vi "thermometer_prac2.vi"() -> ()   [LabVIEW 2020]
panel:
  in  "Skala temperatury":bool
  out "Temperatura [F]":dbl(slide) scale=0.0..100.0
  out "Temperatura [C]":dbl(slide) scale=0.0..100.0
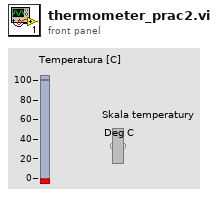
[diagram p1: front panel]
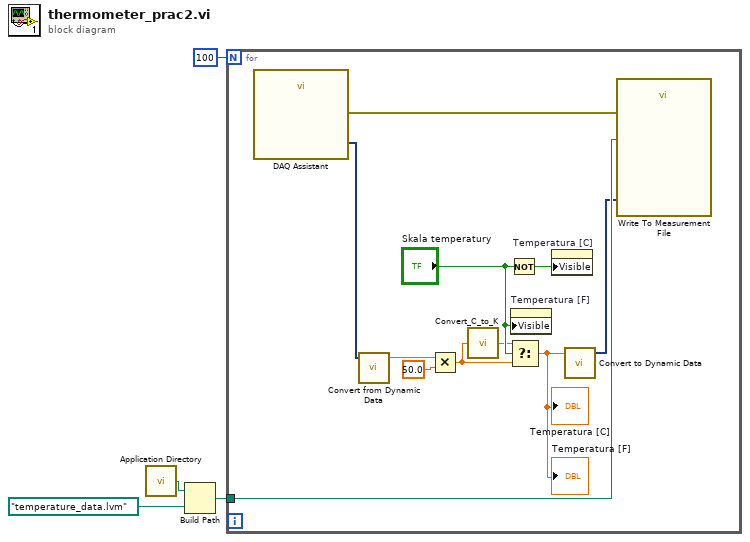
[diagram p0: block diagram]
diagram:
  n1 = call <vilib>:"Application Directory.vi"() -> ("Application Directory"=w3:path)
  n2 = Build Path(base path=w3, name or relative path=path "temperature_data.lvm") -> (appended path=w2:path)
  n3 = for {
    N: 100 -> [_]
    tunnel: w2 -> [w8]
    n4 = call "DAQ Assistant"() -> ("data"=w14:dynamicdata, "error out"=w5:errorcluster)  [unwired: 16 in, 2 out]
    n5 = call "Convert from Dynamic Data"("Dynamic Data Type"=w14) -> ("Scalar"=w13:dbl)  [unwired: 3 in]
    n6 = Multiply(x=w13, y=50.0) -> (x*y=w9:dbl)
    n7 = call "Convert_C_to_K.vi"("deg C"=w9) -> ("deg F"=w10:dbl)
    n8 = Not(x="Skala temperatury") -> (.not. x?=w11:bool)
    n9 = Select(t=w10, s="Skala temperatury", f=w9) -> (s? t:f=w7:dbl)
    "Temperatura [C]" <- w7
    "Temperatura [F]" <- w7
    n10 = property on="Temperatura [F]" class="Slide (strict)"("Visible"="Skala temperatury") -> ()  [unwired: 2 in, 2 out]
    n11 = property on="Temperatura [C]" class="Slide (strict)"("Visible"=w11) -> ()  [unwired: 2 in, 2 out]
    n12 = call "Convert to Dynamic Data"("Double"=w7) -> ("Dynamic Data Type"=w6:dynamicdata)  [unwired: 3 in]
    n13 = call "Write To Measurement File"("Signals"=w6, "error in (no error)"=w5, "Filename"=w8) -> ()  [unwired: 14 in, 3 out]
  }
